vi "Get All Control Values {Variant}__ogtk.vi"(8 "error in (no error)":errorcluster, 10 "controls (FALSE: indicators)":bool, 11 "VI Refnum":refnum<vi>) -> (0 "error out":errorcluster, 2 "All Control Values":cluster{"Name":string, "Variant Data":variant}[](array[cluster]), 3 "VI Refnum dup":refnum<vi>)   [LabVIEW 2018]
doc: "Gets all of the control of indicator values depending on the Boolean input Control. An input of TRUE will return all of the control while an input of FALSE will return all of the indicators.\n\n<b>Note: </b>This VI used to call an IN that is now depreciated. As a result, this VI has become a redundant wrapper.\n\n<b>This VI Is Depreciated</b> \nPlease use \"Invoke Node:Ctrl Val.Get All\" available from the Functions Palette."
panel:
  # "This VI Is Depreciated. \nPlease use \"Invoke Node:Ctrl Val.Get All\" available from the Functions Palette."
  # "Please visit http://www.OpenG.org to learn about the\nOpen Source LabVIEW software movement.\n\nNOTICE -- YOU MUST LEAVE THIS NOTICE IN PLACE.  PER THE TERMS OF THE LICENSE BELOW, YOU MAY SUBLICENSE THIS SOFTWARE \nIN ANY WAY THAT DOES NOT CONFLICT WITH THIS LICENSE.\n\n### BSD License (http://www.opensource.org/licenses/bsd-license.php) Begin ###\n \nCopyright (c) 2002, Jean-Pierre Drolet <drolet_jp@hotmail.com>\nCopyright (c) 2002, Jim Kring <jim@jimkring.com>\nCopyright (c) 2011, Jonathon Green <jg@jgcode.net>\n\nAll rights reserved.\n\nRedistribution and use in source and binary forms, with or without modification, are permitted provided that the following conditions are met:\n\n    * Redistributions of source code must retain the above copyright notice, this list of conditions and the following disclaimer.\n    * Redistributions in binary form must reproduce the above copyright notice, this list of conditions and the following disclaimer in the \n       documentation and/or other materials provided with the distribution.\n    * Neither the name of SciWare, James Kring, Inc., nor the names of its contributors may be used to endorse or promote products derived \n       from this software without specific prior written permission.\n\nTHIS SOFTWARE IS PROVIDED BY THE COPYRIGHT HOLDERS AND CONTRIBUTORS \"AS IS\" AND ANY EXPRESS OR IMPLIED WARRANTIES, \nINCLUDING, BUT NOT LIMITED TO, THE IMPLIED WARRANTIES OF MERCHANTABILITY AND FITNESS FOR A PARTICULAR PURPOSE ARE \nDISCLAIMED. IN NO EVENT SHALL THE COPYRIGHT OWNER OR CONTRIBUTORS BE LIABLE FOR ANY DIRECT, INDIRECT, INCIDENTAL,\n SPECIAL, EXEMPLARY, OR CONSEQUENTIAL DAMAGES (INCLUDING, BUT NOT LIMITED TO, PROCUREMENT OF SUBSTITUTE GOODS OR \nSERVICES; LOSS OF USE, DATA, OR PROFITS; OR BUSINESS INTERRUPTION) HOWEVER CAUSED AND ON ANY THEORY OF LIABILITY, \nWHETHER IN CONTRACT, STRICT LIABILITY, OR TORT (INCLUDING NEGLIGENCE OR OTHERWISE) ARISING IN ANY WAY OUT OF THE USE \nOF THIS SOFTWARE, EVEN IF ADVISED OF THE POSSIBILITY OF SUCH DAMAGE.\n\n### BSD License End ###"
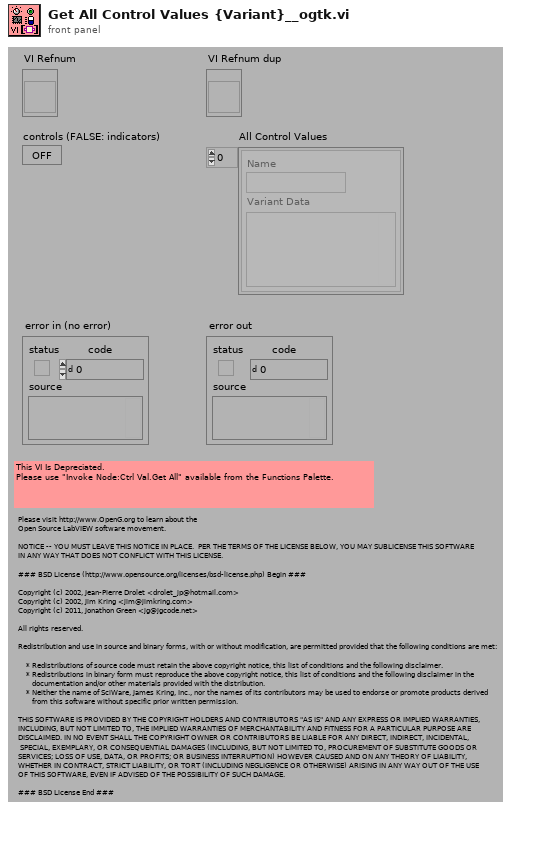
[diagram p1: front panel]
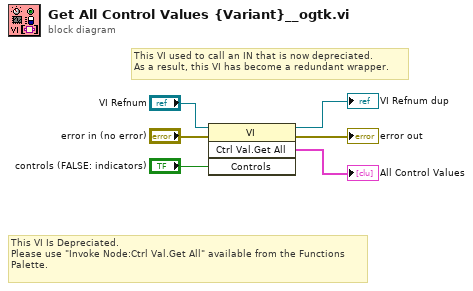
[diagram p0: block diagram]
diagram:
  # "This VI Is Depreciated. \nPlease use \"Invoke Node:Ctrl Val.Get All\" available from the Functions Palette."
  # "This VI used to call an IN that is now depreciated.\nAs a result, this VI has become a redundant wrapper."
  n1 = invoke class="VI" method="Ctrl Val.Get All"(reference="VI Refnum", error in="error in (no error)", "Controls"="controls (FALSE: indicators)") -> (reference out=→"VI Refnum dup":refnum<vi>, error out=→"error out":errorcluster, "Get All Control Values Variant"=→"All Control Values":cluster{"Name":string, "Variant Data":variant}[])  [unwired: 1 in, 1 out]
